vi "TIFFStream Write.vi"(7 "File data":T1, 8 "error in (no error)":errorcluster, 9 "Last image in file?":bool, 10 "IFD Offset":u32, 11 "Image data reference":refnum<data-value>) -> (0 "error out":errorcluster, 2 "Next IFD Offset":u32)   [LabVIEW 2015]
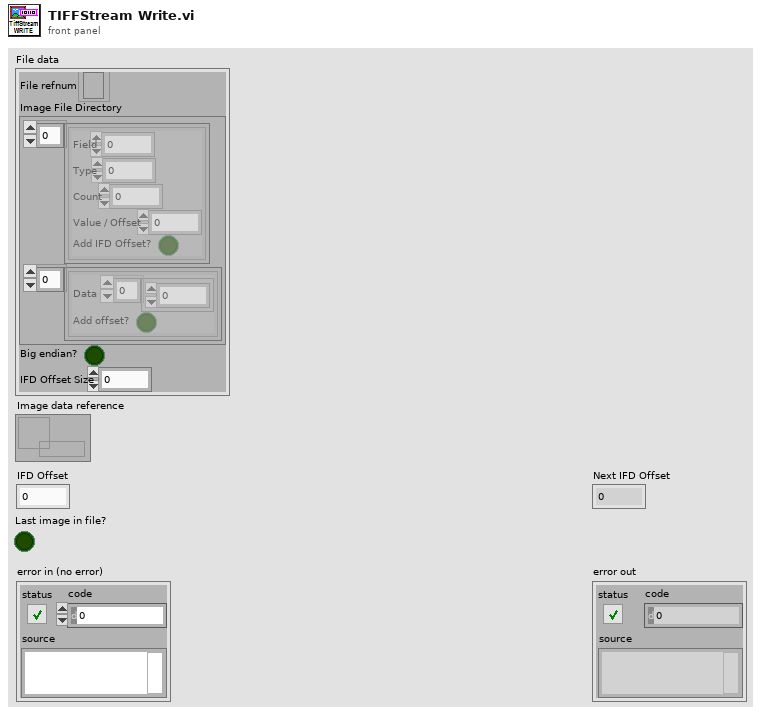
[diagram p1: front panel]
types:
  T1 = cluster{"File refnum":refnum<file>, "Image File Directory":cluster{cluster{"Field":u16, "Type":u16, "Count":u32, "Value / Offset":u32, "Add IFD Offset?":bool}[], cluster{"Data":u32[], "Add offset?":bool}[]}, "Big endian?":bool, "IFD Offset Size":u32}
  T2 = enum16{"big-endian, network order", "native, host order", "little-endian"}
  T3 = cluster{cluster{"Field":u16, "Type":u16, "Count":u32, "Value / Offset":u32, "Add IFD Offset?":bool}[], cluster{"Data":u32[], "Add offset?":bool}[]}
  T4 = cluster{"Field":u16, "Type":u16, "Count":u32, "Value / Offset":u32, "Add IFD Offset?":bool}[]
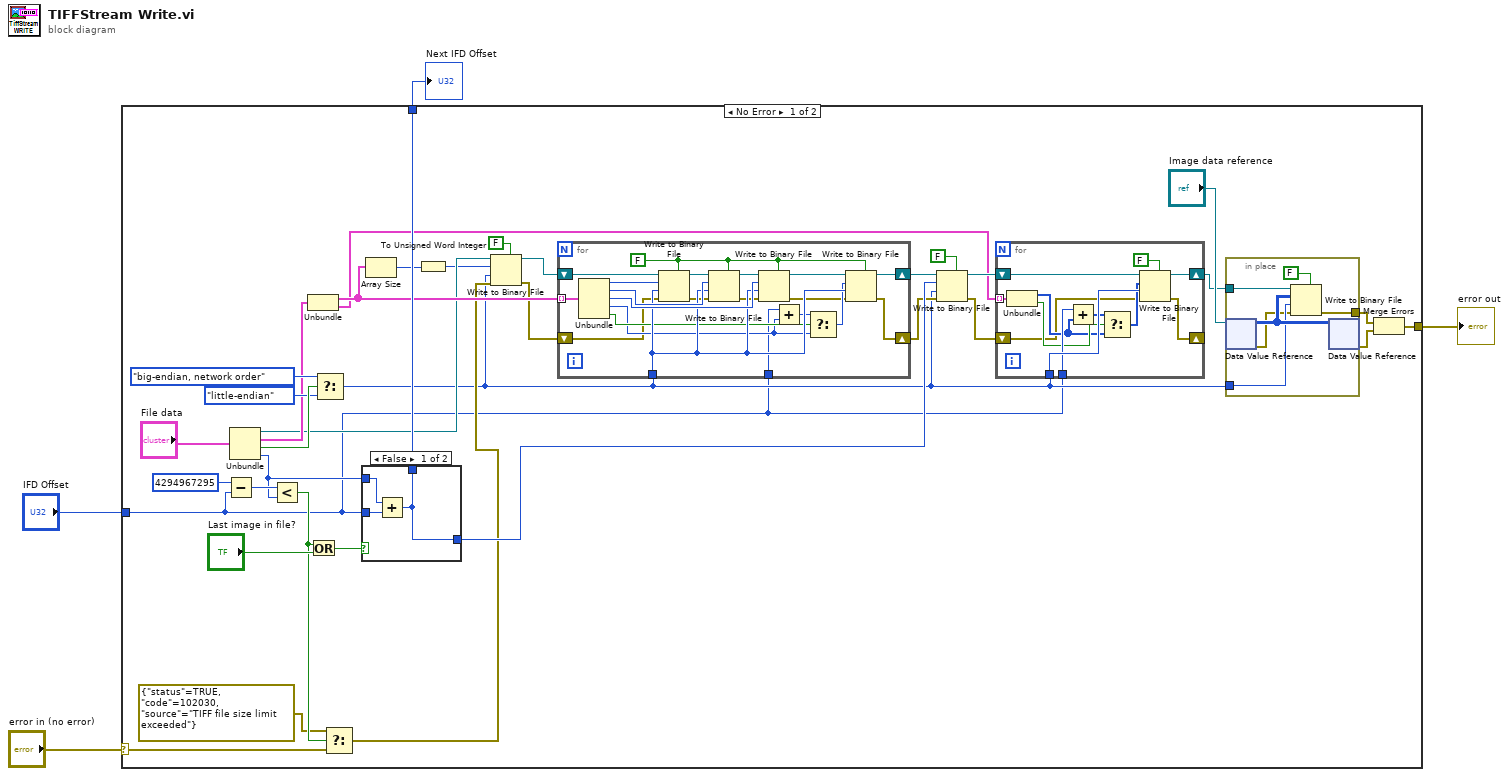
[diagram p0: block diagram]
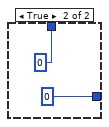
[diagram p2: hidden frame]
diagram:
  n1 = case shown="No Error" "error in (no error)" {
    selector: "error in (no error)" -> [w27 w85]
    tunnel: [w35 w85] -> w4
    tunnel: [w34 w86] -> w3
    tunnel: "IFD Offset" -> [w6 w86]
    frame No Error {
      n2 = Subtract(x=u32 4294967295 ("IFD Offset"), y=w6) -> (x-y=w30:u32)
      n3 = Unbundle("File data") -> ("File refnum"=w18:refnum<file>, "Image File Directory"=w23:T3, "Big endian?"=w40:bool, "IFD Offset Size"=w29:u32)
      n4 = Less?(x=w30, y=w29) -> (x < y?=w28:bool)
      n5 = Unbundle(w23) -> (w20:T4, w9:cluster{"Data":u32[], "Add offset?":bool}[])
      n6 = Or(x=w28, y="Last image in file?") -> (x .or. y?=w33:bool)
      n7 = Select(t=T2."big-endian, network order" ("byte order (0:big-endian, network order)"), s=w40, f=T2."little-endian" ("byte order (0:big-endian, network order)")) -> (s? t:f=w7:T2)
      n8 = Select(t=errorcluster {"status"=TRUE, "code"=102030, "source"="TIFF file size limit exceeded"} ("error IO"), s=w28, f=w27) -> (s? t:f=w14:errorcluster)
      n9 = case shown="False" w33 {
        tunnel: w6 -> [w76 _]
        tunnel: [w74 u32 0] -> w22
        tunnel: w29 -> [w75 _]
        tunnel: [w74 u32 0] -> w34
        frame False {
          n10 = Add(x=w75, y=w76) -> (x+y=w74:u32)
        }
        frame True {
        }
      }
      n11 = Array Size(array=w20) -> (size(s)=w19:i32)
      n12 = To Unsigned Word Integer(number=w19) -> (unsigned 16bit integer=w16:u16)
      n13 = Write to Binary File(file (use dialog)=w18, data=w16, error in=w14, 5:FALSE ("prepend array or string size? (T)"), 9:w7) -> (refnum out=w17:refnum<file>, error out=w15:errorcluster)  [unwired: 1 in, 1 out]
      n14 = for {
        tunnel: w20 -> [w73] mode=indexing
        tunnel: w7 -> [w64]
        tunnel: w6 -> [w59]
        shift-right: [w54] -> w11
        shift-left: w15 -> [w55]
        shift-right: [w53] -> w12
        shift-left: w17 -> [w67]
        w66 = FALSE ("prepend array or string size? (T)")
        n15 = Unbundle(w73) -> ("Field"=w72:u16, "Type"=w70:u16, "Count"=w68:u32, "Value / Offset"=w60:u32, "Add IFD Offset?"=w63:bool)
        n16 = Write to Binary File(file (use dialog)=w67, data=w72, error in=w55, 5:w66, 9:w64) -> (refnum out=w71:refnum<file>, error out=w58:errorcluster)  [unwired: 1 in, 1 out]
        n17 = Write to Binary File(file (use dialog)=w71, data=w70, error in=w58, 5:w66, 9:w64) -> (refnum out=w69:refnum<file>, error out=w57:errorcluster)  [unwired: 1 in, 1 out]
        n18 = Write to Binary File(file (use dialog)=w69, data=w68, error in=w57, 5:w66, 9:w64) -> (refnum out=w65:refnum<file>, error out=w56:errorcluster)  [unwired: 1 in, 1 out]
        n19 = Add(x=w59, y=w60) -> (x+y=w61:u32)
        n20 = Select(t=w61, s=w63, f=w60) -> (s? t:f=w62:u32)
        n21 = Write to Binary File(file (use dialog)=w65, data=w62, error in=w56, 5:w66, 9:w64) -> (refnum out=w53:refnum<file>, error out=w54:errorcluster)  [unwired: 1 in, 1 out]
      }
      n22 = Write to Binary File(file (use dialog)=w12, data=w22, error in=w11, 5:FALSE ("prepend array or string size? (T)"), 9:w7) -> (refnum out=w10:refnum<file>, error out=w8:errorcluster)  [unwired: 1 in, 1 out]
      n23 = for {
        tunnel: w9 -> [w52] mode=indexing
        tunnel: w7 -> [w50]
        tunnel: w6 -> [w47]
        shift-right: [w46] -> _
        shift-left: w8 -> [w43]
        shift-right: [w41] -> w5
        shift-left: w10 -> [w42]
        n24 = Unbundle(w52) -> ("Data"=w44:u32[], "Add offset?"=w45:bool)
        n25 = Add(x=w47, y=w44) -> (x+y=w48:u32[])
        n26 = Select(t=w48, s=w45, f=w44) -> (s? t:f=w49:u32[])
        n27 = Write to Binary File(file (use dialog)=w42, data=w49, error in=w43, 5:FALSE ("prepend array or string size? (T)"), 9:w50) -> (refnum out=w41:refnum<file>, error out=w46:errorcluster)  [unwired: 1 in, 1 out]
      }
      n28 = in-place {
        in-place-border: w5 -> [w80]
        in-place-border: w7 -> [w83]
        in-place-border: [w81] -> w37
        n29 = in-place-dvr #1("Image data reference") -> (w84:u16[][], w79:errorcluster)
        n30 = Write to Binary File(file (use dialog)=w80, data=w84, error in=w79, 5:FALSE ("prepend array or string size? (T)"), 9:w83) -> (error out=w81:errorcluster)  [unwired: 1 in, 2 out]
        n31 = in-place-dvr #1(w84) -> (w36:errorcluster)  [unwired: 1 out]
      }
      n32 = Merge Errors(w37, w36) -> (w35:errorcluster)
    }
    frame Error {
    }
  }
  "error out" <- w4
  "Next IFD Offset" <- w3
